vi "通过控件名获取控件引用.vi"(8 "控件名数组":string[](array[string]), 10 "错误输入（无错误）":errorcluster, 11 "VI引用":refnum<vi>) -> (0 "控件引用输出":refnum<vi>[](array[refnum]), 2 "错误输出":errorcluster, 3 "VI引用o":refnum<vi>)   [LabVIEW 2017]
panel:
  out "被引用VI路径":path
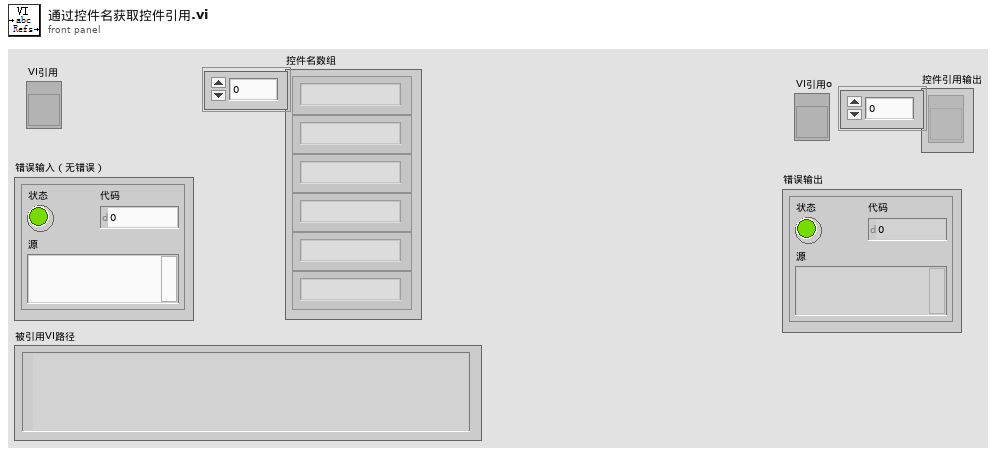
[diagram p1: front panel]
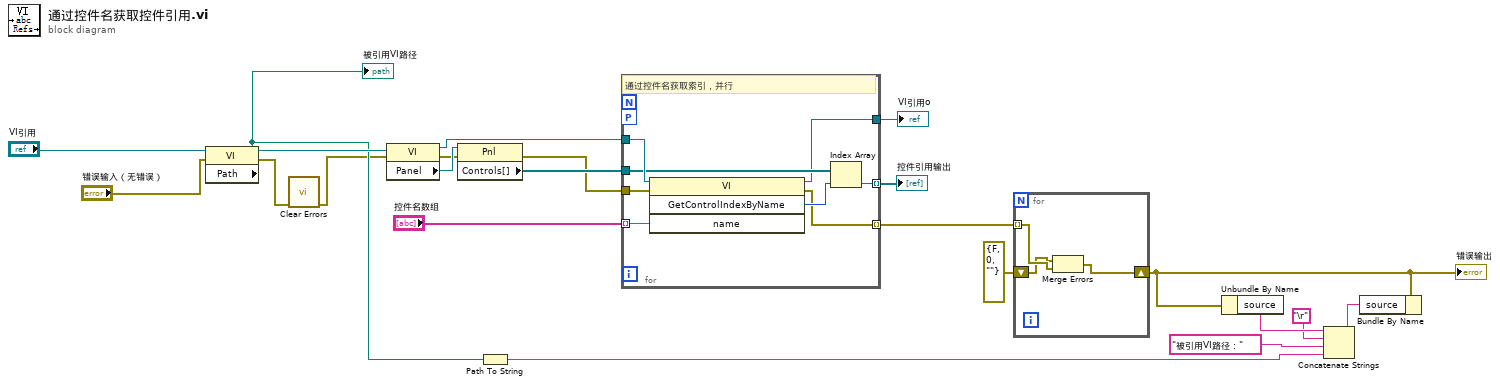
[diagram p0: block diagram]
diagram:
  n1 = property class="VI"(reference="VI引用", error in="错误输入（无错误）") -> (reference out=w15:refnum<vi>, error out=w13:errorcluster, "Path"=w9:path)
  "被引用VI路径" <- w9
  n2 = call <vilib>:"Clear Errors.vi"("error in (no error)"=w13) -> ("error out"=w1:errorcluster)  [unwired: 5 in, 1 out]
  n3 = property class="VI"(reference=w15, error in=w1) -> (reference out=w20:refnum<vi>, error out=w21:errorcluster, "Panel"=w22:refnum<vi>)
  n4 = property class="Pnl"(reference=w22, error in=w21) -> (error out=w10:errorcluster, "Controls[]"=w19:refnum<vi>[])  [unwired: 1 out]
  n5 = Path To String(path=w9) -> (string=w8:string)
  n6 = for "For循环" {
    workers-P: _ -> [_]
    tunnel: w20 -> [w30]
    tunnel: "控件名数组" -> [w29] mode=indexing
    tunnel: w19 -> [w28]
    tunnel: [w26] -> w18 mode=indexing
    tunnel: [w25] -> w17
    tunnel: [w24] -> w11 mode=indexing
    tunnel: w10 -> [w23]
    # "通过控件名获取索引，并行"
    n7 = invoke class="VI" method="GetControlIndexByName"(reference=w30, error in=w23, "name"=w29) -> (reference out=w25:refnum<vi>, error out=w24:errorcluster, "GetControlIndexByName"=w27:i32)  [unwired: 1 in, 1 out]
    n8 = Index Array(array=w28, index=w27) -> (element=w26:refnum<vi>)
  }
  "控件引用输出" <- w18
  "VI引用o" <- w17
  n9 = for {
    tunnel: w11 -> [w33] mode=indexing
    shift-right: [w31] -> w2
    shift-left: errorcluster {"status"=FALSE, "code"=0, "source"=""} ("error IO") -> [w32]
    n10 = Merge Errors(w32, w33) -> (w31:errorcluster)
  }
  "错误输出" <- w2
  n11 = Unbundle By Name(w2) -> ("source"=w7:string)
  n12 = Concatenate Strings(w7, "\r", "被引用VI路径：" ("字符串"), w8) -> (w4:string)
  n13 = Bundle By Name(cluster=w2, "source"=w4) -> ()  [unwired: 1 out]
